vi "Read num1.vi"(8 "error in (no error)":errorcluster, 11 "POffset in":refnum<class "POffset.lvclass">) -> (0 "error out":errorcluster, 2 "num1":T1, 3 "POffset out":refnum<class "POffset.lvclass">)   [LabVIEW 2014, in "TCSDataDefinitions.lvlib" / "TCSCommand.lvlib" / "POriginCommands.lvlib" / "POffset.lvclass"]
uses:
  POffset.lvclass
  OffsetCommands/OffsetDef/Enumerations/Num1Types.ctl
  POffset.lvclass/POffset.ctl
  OffsetCommands/OffsetCommands.lvlib
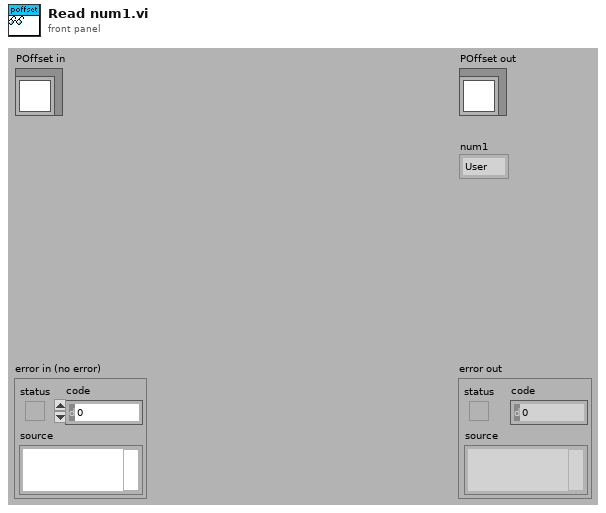
[diagram p1: front panel]
types:
  T1 = typedef "TCSDataDefinitions.lvlib/TCSCommand.lvlib/OffsetCommands.lvlib/Num1Types.ctl" = enum16{"User", "Handset"}
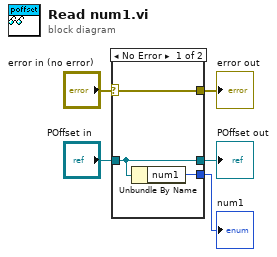
[diagram p0: block diagram]
diagram:
  n1 = case shown="No Error" "error in (no error)" {
    selector: "error in (no error)" -> [w8 w9]
    tunnel: [w8 w9] -> w4
    tunnel: [w7 w10] -> w2
    tunnel: "POffset in" -> [w7 w10]
    tunnel: [w6 _] -> w1
    frame No Error {
      n2 = Unbundle By Name(w7) -> ("num1"=w6:T1)
    }
    frame Error {
    }
  }
  "error out" <- w4
  "POffset out" <- w2
  "num1" <- w1
